vi "N05_Incrementer.vi"() -> ()   [LabVIEW 2023]
panel:
  out "Meeter Out of Loop":dbl(knob) scale=-10.0..180.0
  out "Meter In Loop":dbl(knob) scale=-10.0..180.0
  in  "Down":bool
  in  "Up":bool
  # "Servos use position control between 0 and 170 degrees\nShow the result using a meter with a scale of -10 to 180\nPut one meeter in the while loop and one meeter out of the while loop.\n\nRequirements:\n- I want to use two buttons, up button and down button, to rotate a servo \n- When the up button is pressed increment the position command for the servo\n- When the down button is pressed, decrement the position command for the servo\n- The output is limited between 0 and 170"
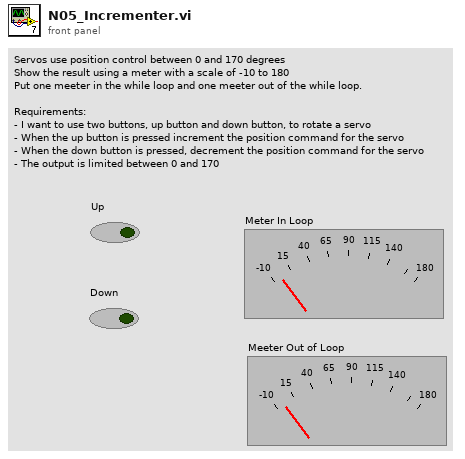
[diagram p1: front panel]
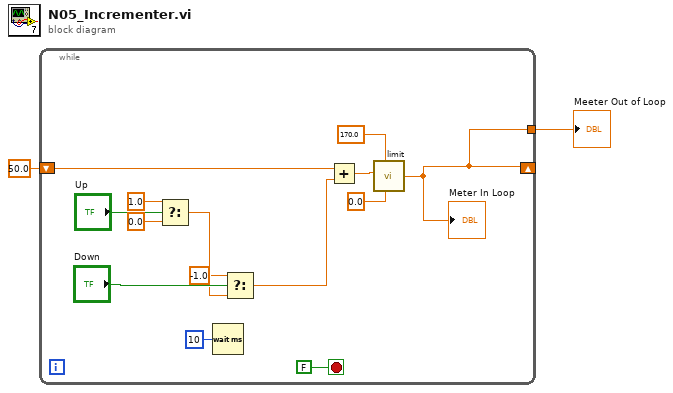
[diagram p0: block diagram]
diagram:
  n1 = while {
    shift-right: [w5] -> _
    shift-left: 50.0 ("t") -> [w8]
    tunnel: [w5] -> w1
    stop <- FALSE stop-if-true
    n2 = Select(t=1.0, s="Up", f=0.0) -> (s? t:f=w12:dbl)
    n3 = Wait (ms)(milliseconds to wait=u32 10) -> ()  [unwired: 1 out]
    n4 = Select(t=-1.0, s="Down", f=w12) -> (s? t:f=w7:dbl)
    n5 = Add(x=w8, y=w7) -> (x+y=w6:dbl)
    n6 = call "limit.vi"("Lower_Limit"=0.0, "Upper_Limit"=170.0, "Input"=w6) -> ("Output"=w5:dbl)  [unwired: 3 in]
    "Meter In Loop" <- w5
  }
  "Meeter Out of Loop" <- w1
